vi "Optical Flow.vi"() -> ()   [LabVIEW 2017]
doc: "This example shows use the Horn Schunck and Lucas Kanade methods to compute dense optical (motion) flow information in a sequence of images. The VI reads the frames and computes the optical flow between consecutive frames."
uses:
  <vilib>/vision/NI_Vision_Development_Module.lvlib
panel:
  in  "Optical Flow Algorithm":enum32{"Horn Schunck", "Lucas Kanade"}(radio)
  out "Image":T1(plugin-control)
  in  "Delay (s.)":dbl(slide)=0.25 scale=0.0..1.5
  out "Progress Bar":i32(slide) max=49 scale=0.0..49.0
  in  "Stop":bool
  # "Overview: Demonstrate the use of the Optical Flow algorithm of Vision Development Module.\nRequirements: Vision Development Module\nInstructions:\nRun the VI."
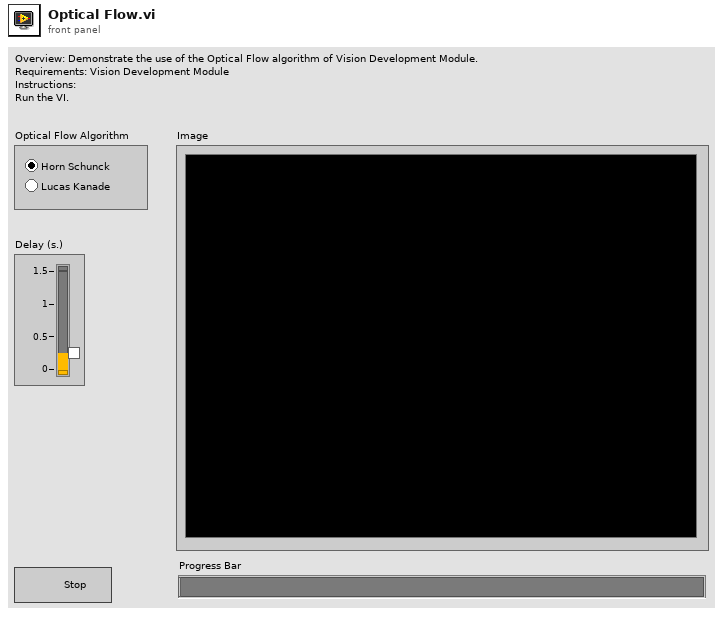
[diagram p1: front panel]
types:
  T1 = typedef "IMAQ Image.ctl" = refnum<image>
  T2 = typedef "Image Type" = u32
  T3 = cluster{"Type":enum16{"Invalid", "Iterations", "Epsilon", "Both"}, "Max. Iterations":i32, "Epsilon":dbl}
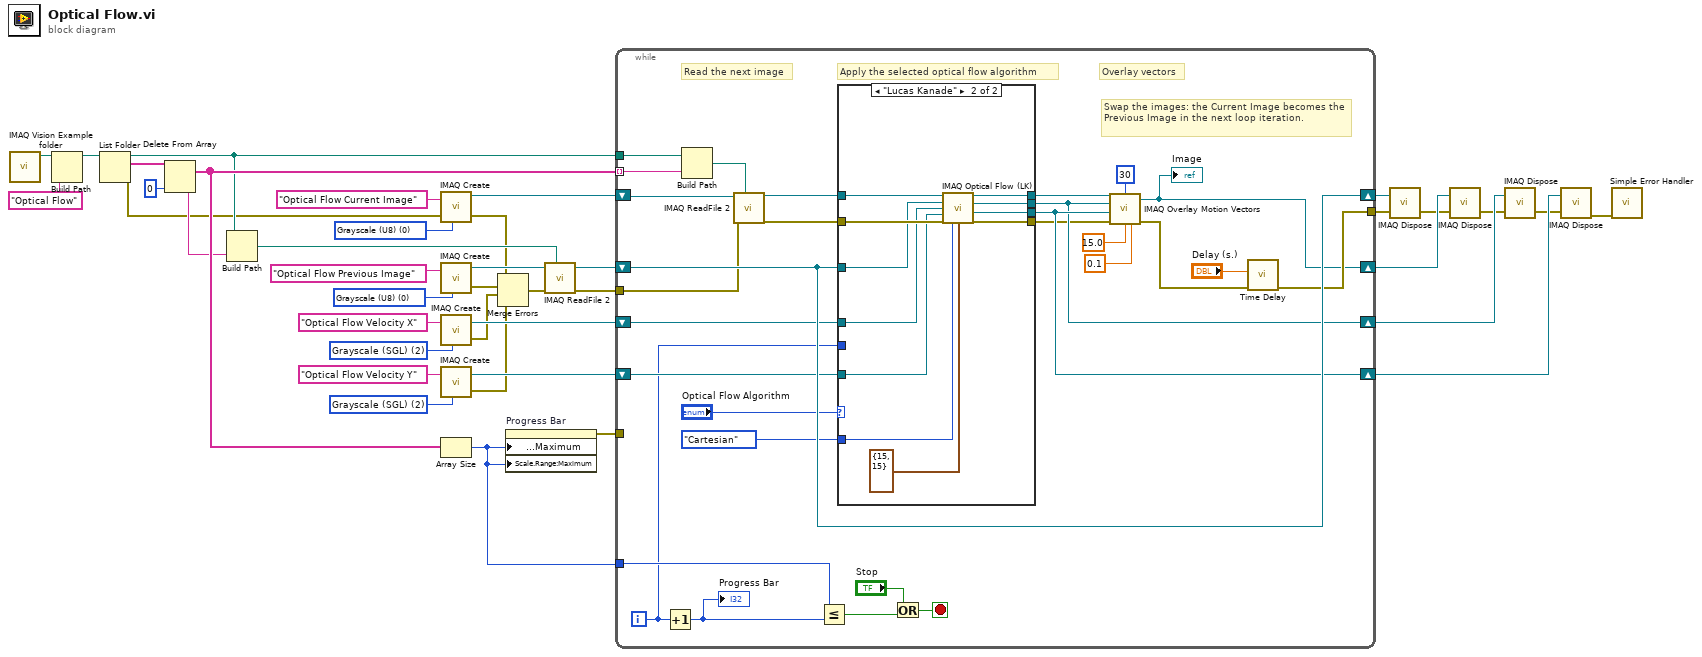
[diagram p0: block diagram]
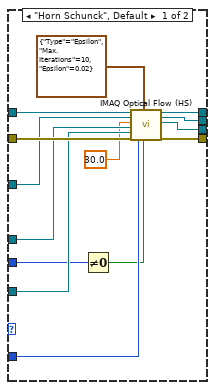
[diagram p2: hidden frame]
diagram:
  w14 = T2 2 items=["Grayscale (U8)", "Grayscale (I16)", "Grayscale (SGL)", "Complex (CSG)", "RGB (U32)", "HSL (U32)", "RGB (U64)", "Grayscale (U16)"] ("Image Type")
  w15 = T2 0 items=["Grayscale (U8)", "Grayscale (I16)", "Grayscale (SGL)", "Complex (CSG)", "RGB (U32)", "HSL (U32)", "RGB (U64)", "Grayscale (U16)"] ("Image Type")
  w31 = T2 0 items=["Grayscale (U8)", "Grayscale (I16)", "Grayscale (SGL)", "Complex (CSG)", "RGB (U32)", "HSL (U32)", "RGB (U64)", "Grayscale (U16)"] ("Image Type")
  w33 = T2 2 items=["Grayscale (U8)", "Grayscale (I16)", "Grayscale (SGL)", "Complex (CSG)", "RGB (U32)", "HSL (U32)", "RGB (U64)", "Grayscale (U16)"] ("Image Type")
  n1 = call "IMAQ Vision Example folder.vi"() -> ("Example Image Path"=w2:path)  [unwired: 11 in]
  n2 = Build Path(base path=w2, name or relative path="Optical Flow") -> (appended path=w16:path)
  n3 = List Folder(path=w16) -> (path out=w19:path, filenames=w23:string[], error out=w13:errorcluster)  [unwired: 1 in, 3 out]
  n4 = Delete From Array(array=w23, index=0) -> (deleted portion=w18:string, array with subset deleted=w20:string[])  [unwired: 1 in]
  n5 = Build Path(base path=w19, name or relative path=w18) -> (appended path=w17:path)
  n6 = call "IMAQ Create"("Image Name"="Optical Flow Current Image", "Image Type"=w31, "error in (no error)"=w13) -> ("New Image"=w39:T1, "error out"=w12:errorcluster)  [unwired: 1 in, 1 out]
  n7 = call "IMAQ Create"("Image Name"="Optical Flow Previous Image", "Image Type"=w15) -> ("New Image"=w26:T1, "error out"=w10:errorcluster)  [unwired: 2 in, 1 out]
  n8 = call "IMAQ Create"("Image Name"="Optical Flow Velocity X", "Image Type"=w33) -> ("New Image"=w36:T1, "error out"=w9:errorcluster)  [unwired: 2 in, 1 out]
  n9 = call "IMAQ Create"("Image Name"="Optical Flow Velocity Y", "Image Type"=w14) -> ("New Image"=w32:T1, "error out"=w11:errorcluster)  [unwired: 2 in, 1 out]
  n10 = Array Size(array=w20) -> (size(s)=w21:i32)
  n11 = Merge Errors(w12, w10, w9, w11) -> (w8:errorcluster)
  n12 = property on="Progress Bar" class="Slide (strict)"("Data Entry Limits:Maximum"=w21, "Scale.Range:Maximum"=w21) -> (error out=w38:errorcluster)  [unwired: 2 in, 1 out]
  n13 = call "IMAQ ReadFile 2"("File Path"=w17, "error in (no error)"=w8, "Image"=w26) -> ("error out"=w25:errorcluster, "Image Out"=w24:T1)  [unwired: 4 in, 3 out]
  n14 = while {
    tunnel: [w57] -> w7
    tunnel: w21 -> [w68]
    tunnel: w38 -> [_]
    shift-right: [w58] -> w29
    shift-left: w36 -> [w66]
    shift-right: [w64] -> w28
    shift-left: w32 -> [w65]
    shift-right: [w56] -> w27
    shift-left: w24 -> [w67]
    tunnel: w25 -> [w62]
    tunnel: w19 -> [w61]
    tunnel: w20 -> [w60] mode=indexing
    shift-right: [w67] -> w30
    shift-left: w39 -> [w69]
    i -> [w59]
    stop <- w41 stop-if-true
    # "Swap the images: the Current Image becomes the Previous Image in the next loop iteration."
    # "Overlay vectors"
    # "Read the next image"
    # "Apply the selected optical flow algorithm"
    n15 = Increment(x=w59) -> (x+1=w63:i32)
    "Progress Bar" <- w63
    n16 = Build Path(base path=w61, name or relative path=w60) -> (appended path=w46:path)
    n17 = call "IMAQ ReadFile 2"("File Path"=w46, "error in (no error)"=w62, "Image"=w69) -> ("error out"=w52:errorcluster, "Image Out"=w51:T1)  [unwired: 4 in, 3 out]
    n18 = Less Or Equal?(x=w68, y=w63) -> (x <= y?=w54:bool)
    n19 = case shown="\"Lucas Kanade\"" "Optical Flow Algorithm" {
      tunnel: w52 -> [w83 w94]
      tunnel: w51 -> [w82 w89]
      tunnel: w66 -> [w80 w87]
      tunnel: w65 -> [w79 w86]
      tunnel: [w77 w93] -> w50
      tunnel: [w76 w92] -> w49
      tunnel: [w75 w90] -> w64
      tunnel: [w74 w91] -> w58
      tunnel: w67 -> [w73 w88]
      tunnel: enum16{"Cartesian", "Polar"}."Cartesian" ("Velocity Representation") -> [w72 w84]
      tunnel: w59 -> [w70 _]
      frame "Horn Schunck", Default {
        n20 = Not Equal To 0?(x=w70) -> (x != 0?=w71:bool)
        n21 = call "IMAQ Optical Flow (HS)"("Current Frame"=w82, "Previous Frame"=w73, "Smoothing Parameter"=sgl 30.0, "Velocity Component 1 In"=w80, "Velocity Component 2 In"=w79, "error in (no error)"=w83, "Velocity Representation"=w72, "Stopping Criteria"=T3 {"Type"=enum."Epsilon", "Max. Iterations"=10, "Epsilon"=0.02}, "Use Previous"=w71) -> ("Current Frame Out (dup)"=w76:T1, "Velocity Component 1 Out"=w74:T1, "Velocity Component 2 Out"=w75:T1, "error out"=w77:errorcluster)  [unwired: 1 in, 6 out]
      }
      frame "Lucas Kanade" {
        n22 = call "IMAQ Optical Flow (LK)"("Current Frame"=w89, "Previous Frame"=w88, "Velocity Component 1 In"=w87, "Velocity Component 2 In"=w86, "error in (no error)"=w94, "Velocity Representation"=w84, "Window Size (15x15)"=cluster{"Size X":i32, "Size Y":i32} {"Size X"=15, "Size Y"=15}) -> ("Current Frame Out (dup)"=w92:T1, "Velocity Component 1 Out"=w91:T1, "Velocity Component 2 Out"=w90:T1, "error out"=w93:errorcluster)  [unwired: 1 in, 4 out]
      }
    }
    n23 = Or(x="Stop", y=w54) -> (x .or. y?=w41:bool)
    n24 = call "IMAQ Overlay Motion Vectors"("Image"=w49, "Step Size"=30, "Velocity Component 1"=w58, "Velocity Component 2"=w64, "error in (no error)"=w50, "Scale"=15.0, "Threshold"=0.1) -> ("Image Out"=w56:T1, "error out"=w45:errorcluster)  [unwired: 3 in, 4 out]
    "Image" <- w56
    n25 = call "Time Delay"("error in (no error)"=w45, "Delay Time (s)"="Delay (s.)") -> ("error out"=w57:errorcluster)  [unwired: 9 in]
  }
  n26 = call "IMAQ Dispose"("Image"=w30, "error in (no error)"=w7) -> ("error out"=w6:errorcluster)  [unwired: 1 in, 3 out]
  n27 = call "IMAQ Dispose"("Image"=w27, "error in (no error)"=w6) -> ("error out"=w5:errorcluster)  [unwired: 1 in, 3 out]
  n28 = call "IMAQ Dispose"("Image"=w29, "error in (no error)"=w5) -> ("error out"=w4:errorcluster)  [unwired: 1 in, 3 out]
  n29 = call "IMAQ Dispose"("Image"=w28, "error in (no error)"=w4) -> ("error out"=w3:errorcluster)  [unwired: 1 in, 3 out]
  n30 = call <vilib>:"Simple Error Handler.vi"("error in (no error)"=w3) -> ()  [unwired: 1 in, 8 out]
